vi "Convert CDO Module to Slot Configuration.vi"(8 "error in":errorcluster, 9 "module in":refnum<class "Module.lvclass">, 10 "RSI module in":refnum<class "RSI Module.lvclass">, 11 "slot ref in":T1 format="%.0x") -> (0 "error out":errorcluster, 3 "slot ref out":T1 format="%.0x")   [LabVIEW 2020, in "Scan Engine Scripting.lvlib"]
uses:
  Scan Engine Scripting.lvlib
  <vilib>/NI VeriStand/Custom Device API/Custom Device Item Ref.ctl
  Modules.lvlibp/RSI Module/RSI Module.lvclass
  Modules/Module/Module.lvclass
  Modules.lvlibp/SD Module/SD Module.lvclass
  C:/jenkins/workspace/ercat-custom-device_release_20.4/Custom Device Source/Modules.lvlibp/RSI Module/RSI Module.lvclass
  <vilib>/NI VeriStand/Custom Device API/Custom Device API.lvlib
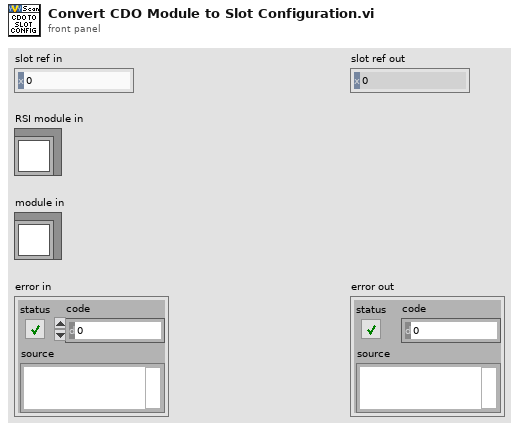
[diagram p1: front panel]
types:
  T1 = typedef "Custom Device API.lvlib/Custom Device Item Ref.ctl" = u64
  T2 = typedef "Scan Engine Scripting.lvlib/Counter Driven Output Mode.lvclass/Drive from Slot.ctl" = enum16{"Slot 1", "Slot 2", "Slot 3", "Slot 4", "Slot 5", "Slot 6", "Slot 7", "Slot 8"}
  T3 = typedef "Scan Engine Scripting.lvlib/counter driven output channel settings.ctl" = cluster{"name":string, "default value":bool, "counter driven state":T4}
  T4 = typedef "Scan Engine Scripting.lvlib/Counter Driven Output Channel.lvclass/Counter Driven State.ctl" = enum16{"Disabled", "Enabled"}
  T5 = typedef "Modules.lvlibp/SD Module.lvclass/CDO.ctl" = cluster{"Drive From Slot":u32, "CDO Channels":T6[]}
  T6 = typedef "Modules.lvlibp/SD Module.lvclass/CDO Channel.ctl" = cluster{"Counter driven enabled":bool}
  T7 = typedef "Modules.lvlibp/Custom Device API.lvlib/Custom Device Item Ref.ctl" = u64
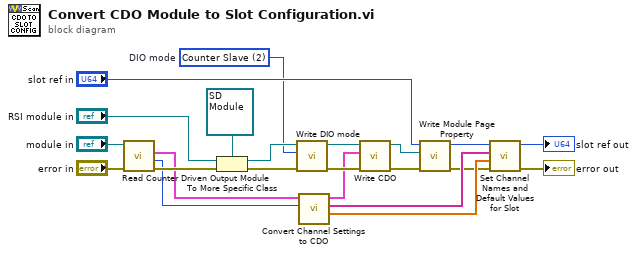
[diagram p0: block diagram]
diagram:
  w1 = u32 2 items=["Normal", "Counter", "Counter Slave", "PWM", "Quadrature"]  # DIO mode
  n1 = call-dynamic "Read Counter Driven Output Module.vi"("error in"="error in", "module in"="module in") -> ("error out"=w7:errorcluster, "drive from slot"=w2:T2, "channel settings"=w3:T3[])  [unwired: 6 in, 1 out]
  n2 = To More Specific Class(target class=refnum<class "SD Module.lvclass"> refnum ("Modules.lvlibp:SD Module.lvclass"), reference="RSI module in", error in=w7) -> (specific class reference=w9:refnum<class "SD Module.lvclass">, error out=w11:errorcluster)
  n3 = call-dynamic "Write DIO mode.vi"("error in (no error)"=w11, "DIO mode"=w1, "SD Module in"=w9) -> ("error out"=w21:errorcluster, "SD Module out"=w22:refnum<class "SD Module.lvclass">)  [unwired: 7 in]
  n4 = call "Convert Channel Settings to CDO.vi"("drive from slot"=w2, "channel settings"=w3) -> ("channel default values"=w20:dbl[], "channel names"=w18:string[], "CDO"=w12:T5)  [unwired: 7 in]
  n5 = call-dynamic "Write CDO.vi"("error in (no error)"=w21, "CDO"=w12, "SD Module in"=w22) -> ("error out"=w13:errorcluster, "SD Module out"=w14:refnum<class "SD Module.lvclass">)  [unwired: 7 in]
  n6 = call "Write Module Page Property.vi"("error in (no error)"=w13, "RSI Module"=w14, "Node Ptr In"="slot ref in") -> ("error out"=w15:errorcluster, "Node Ptr Out"=w16:T7)  [unwired: 6 in, 1 out]
  n7 = call "Set Channel Names and Default Values for Slot.vi"("error in"=w15, "default values"=w20, "channel names"=w18, "slot ref in"=w16) -> ("error out"=→"error out":errorcluster, "slot ref out"=→"slot ref out":T1)  [unwired: 6 in]
